vi "Indent Lines in String.vi"(7 "Indentation Character (\"\\s\")":string=" ", 9 "Indent Level":i32, 11 "Lines in":string) -> (3 "Indented Lines out":string)   [LabVIEW 2011]
doc: "Indents all of the lines with a number of Indentation Characters specified by Indent Level. Indentation Character is a space character \"\\s\" by default."
uses:
  <userlib>/_OpenG.lib/string/string.llb/Convert EOLs (String)__ogtk.vi
panel:
  # "Copyright © 2006 James Kring, Inc. All rights reserved.\n\nAuthor: Jim Kring <jim.kring@jameskring.com>\n\nThis library is provided \"AS IS\" , WITHOUT WARRANTIES OR \nCONDITIONS OF ANY KIND, either express or implied.\n\nJames Kring, Inc. -- http://www.jameskring.com"
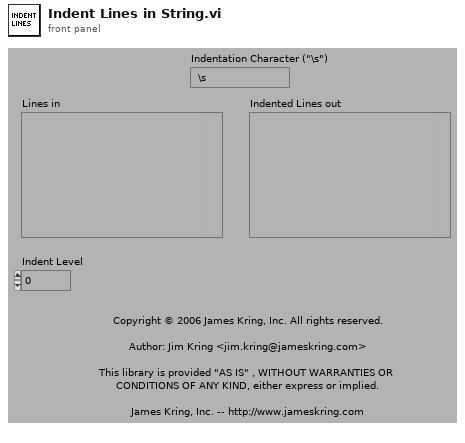
[diagram p1: front panel]
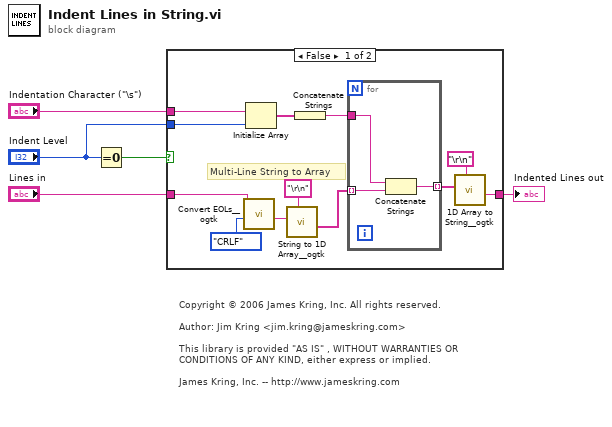
[diagram p0: block diagram]
diagram:
  # "Copyright © 2006 James Kring, Inc. All rights reserved.\n\nAuthor: Jim Kring <jim.kring@jameskring.com>\n\nThis library is provided \"AS IS\" , WITHOUT WARRANTIES OR \nCONDITIONS OF ANY KIND, either express or implied.\n\nJames Kring, Inc. -- http://www.jameskring.com"
  n1 = Equal To 0?(x="Indent Level") -> (x = 0?=w1:bool)
  n2 = case shown="False" w1 {
    tunnel: "Lines in" -> [w7 w21]
    tunnel: "Indentation Character (\"\\s\")" -> [w15 _]
    tunnel: [w12 w21] -> w3
    tunnel: "Indent Level" -> [w11 _]
    frame False {
      # "Multi-Line String to Array"
      n3 = call-poly <userlib>:"Convert EOLs__ogtk.vi"("Convert to:"=enum16{"CR", "LF", "CRLF"}."CRLF", "String in"=w7) -> ("String out"=w9:string)  [unwired: 9 in]
      n4 = Initialize Array(w15, w11) -> (w16:string[])
      n5 = call <userlib>:"String to 1D Array__ogtk.vi"("delimiter (Tab)"="\r\n", "string"=w9) -> ("Array of Strings"=w6:string[])  [unwired: 9 in]
      n6 = Concatenate Strings(w16) -> (w17:string)
      n7 = for {
        tunnel: w6 -> [w20] mode=indexing
        tunnel: w17 -> [w19]
        tunnel: [w18] -> w14 mode=indexing
        n8 = Concatenate Strings(w19, w20) -> (w18:string)
      }
      n9 = call <userlib>:"1D Array to String__ogtk.vi"("delimiter (Tab)"="\r\n", "Array of Strings"=w14) -> ("delimited string"=w12:string)  [unwired: 9 in]
    }
    frame True {
    }
  }
  "Indented Lines out" <- w3
